vi "0.4_кВ_В1.vi"(8 "Time delay":dbl, 9 "Авария ВВОД 1":bool) -> (1 "АВР\nВВОД1 2":bool, 2 "Амперметр 0,4 кВ ВВОД1 2":dbl(knob) scale=0.0..630.0, 3 "Вольтметр 0,4 кВ ВВОД 2":i64(knob) scale=340.0..420.0)   [LabVIEW 2016]
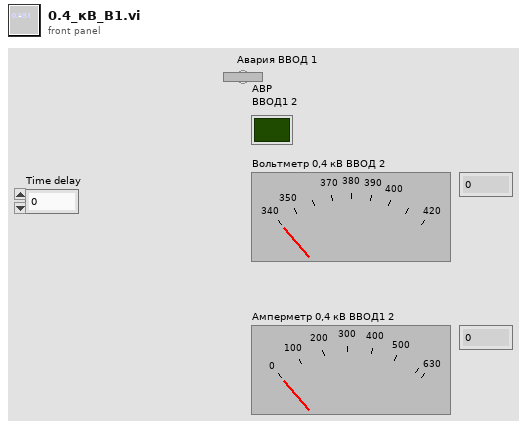
[diagram p1: front panel]
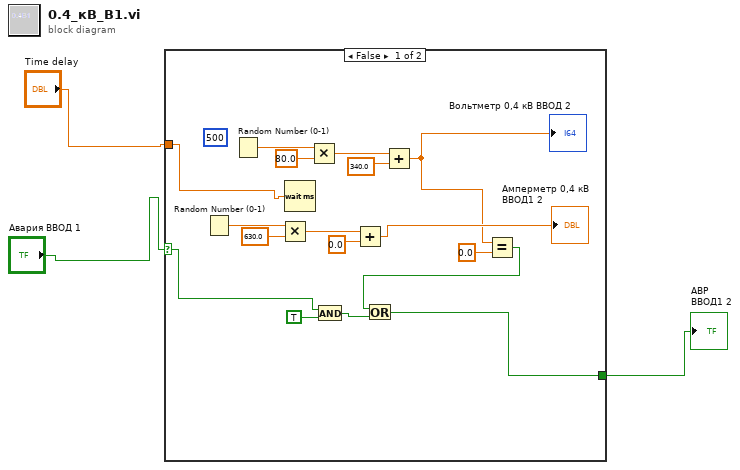
[diagram p0: block diagram]
diagram:
  n1 = case shown="False" "Авария ВВОД 1" {
    selector: "Авария ВВОД 1" -> [w6 w21]
    tunnel: "Time delay" -> [w5 _]
    tunnel: [w4 w21] -> w1
    frame False {
      (unwired) u32 500 ("milliseconds to wait")
      n2 = Random Number (0-1)() -> (number: 0 to 1=w14:dbl)
      n3 = Random Number (0-1)() -> (number: 0 to 1=w10:dbl)
      n4 = Multiply(x=w14, y=630.0) -> (x*y=w16:dbl)
      n5 = Wait (ms)(milliseconds to wait=w5) -> ()  [unwired: 1 out]
      n6 = Multiply(x=w10, y=80.0) -> (x*y=w12:dbl)
      n7 = And(x=w6, y=TRUE) -> (x .and. y?=w19:bool)
      n8 = Add(x=w16, y=0.0) -> (x+y=→"Амперметр 0,4 кВ ВВОД1 2":dbl)
      n9 = Add(x=w12, y=340.0) -> (x+y=w7:dbl)
      "Вольтметр 0,4 кВ ВВОД 2" <- w7
      n10 = Equal?(x=w7, y=0.0) -> (x = y?=w20:bool)
      n11 = Or(x=w20, y=w19) -> (x .or. y?=w4:bool)
    }
    frame True {
    }
  }
  "АВР\nВВОД1 2" <- w1
